vi "cmd.vi"() -> ()   [LabVIEW 2016]
panel:
  in  "stop":bool
  out "Array 2":dbl[](array[numeric])=[45852.0, 295948.0]
  out "error out":errorcluster
  out "return code":i32
  out "standard error":string
  out "standard output":string="EndNote.exe                   4208 Console                    1     45,852 K\r\nLabVIEW.exe                  13532 Console                    1    295,948 K\r\n"
  in  "command line (utility)":string="cmd /c tasklist | findstr \"LabVIEW VRM\" "
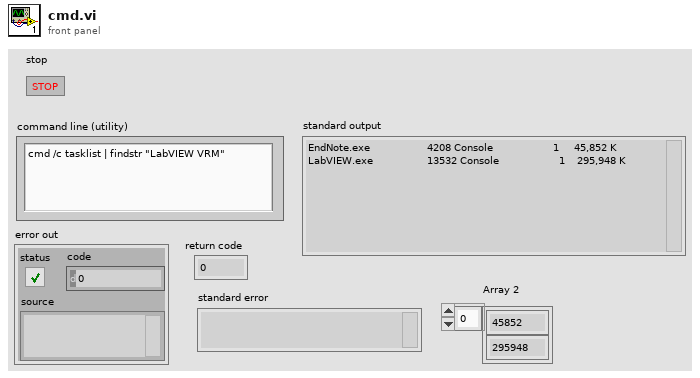
[diagram p1: front panel]
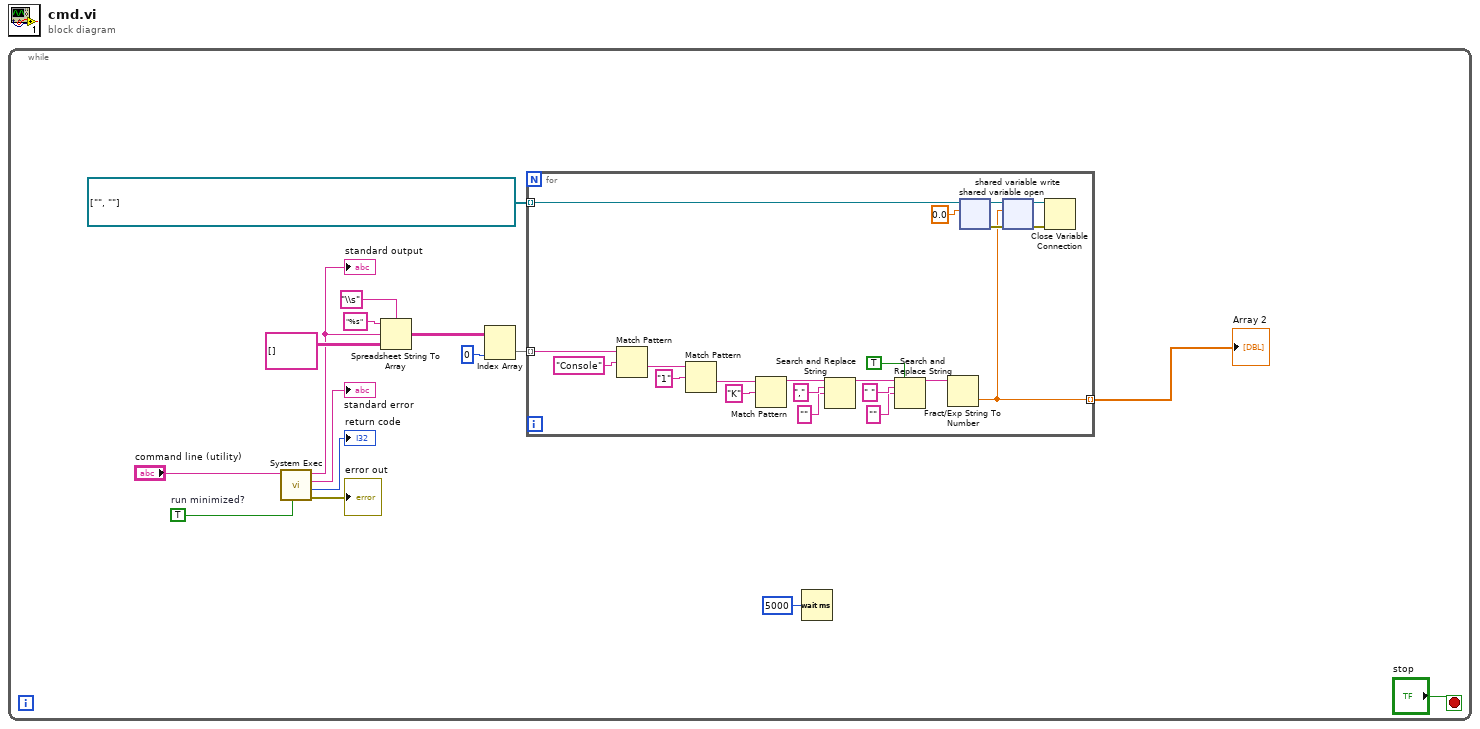
[diagram p0: block diagram]
diagram:
  n1 = while {
    stop <- "stop" stop-if-true
    w15 = TRUE  # run minimized?
    n2 = call <vilib>:"System Exec.vi"("run minimized? (F)"=w15, "command line"="command line (utility)") -> ("error out"=→"error out":errorcluster, "return code"=→"return code":i32, "standard error"=→"standard error":string, "standard output"=w10:string)  [unwired: 4 in, 2 out]
    "standard output" <- w10
    n3 = Spreadsheet String To Array(delimiter (Tab)="\\s", format string="%s", spreadsheet string=w10, array type (2D Dbl)=string[][] []) -> (array=w8:string[][])
    n4 = Index Array(array=w8, index (col)=0 ("disabled index (col)")) -> (element=w5:string[])  [unwired: 1 in]
    n5 = for {
      tunnel: w5 -> [w37] mode=indexing
      tunnel: [w18] -> w4 mode=indexing
      tunnel: refnum<k21>[] ["", ""] -> [w17] mode=indexing
      n6 = Match Pattern(string=w37, regular expression="Console") -> (after substring=w34:string)  [unwired: 1 in, 3 out]
      n7 = Match Pattern(string=w34, regular expression="1") -> (after substring=w32:string)  [unwired: 1 in, 3 out]
      n8 = Match Pattern(string=w32, regular expression="K") -> (before substring=w31:string)  [unwired: 1 in, 3 out]
      n9 = Search and Replace String(input string=w31, search string=",", replace string="" ("replace string (\"\")")) -> (result string=w26:string)  [unwired: 5 in, 3 out]
      n10 = Search and Replace String(replace all?=TRUE ("replace all? (F)"), input string=w26, search string=" ", replace string="" ("replace string (\"\")")) -> (result string=w24:string)  [unwired: 4 in, 3 out]
      n11 = Fract/Exp String To Number(string=w24) -> (number=w18:dbl)  [unwired: 3 in, 1 out]
      n12 = shared-variable-open(w17, 0.0) -> (w22:refnum<k21>, w21:errorcluster)  [unwired: 2 in]
      n13 = shared-variable-write(w22, w21, w18) -> (w23:refnum<k21>, w20:errorcluster)
      n14 = Close Variable Connection(8:w20, 11:w23) -> ()  [unwired: 1 out]
    }
    "Array 2" <- w4
    n15 = Wait (ms)(milliseconds to wait=u32 5000) -> ()  [unwired: 1 out]
  }
